vi "SendCom.vi"(8 "error in (no error)":errorcluster, 9 "data":variant, 10 "Command":T1="CONTROL:DAQmxConnect", 11 "Control in":refnum<class "Control-Server.lvclass">) -> (0 "error out":errorcluster, 3 "Control out":refnum<class "Control-Server.lvclass">)   [LabVIEW 2020, in "Control-Server.lvclass"]
uses:
  Control-Server.lvclass
  C:/dev/TRANCON/Classes/GeneralFunctionality/GeneralFunctionality.lvclass
  dependecies/ControlsVIs/Clusters-def/SERVER-Commands.ctl
  dependecies/ControlsVIs/Clusters-def/Message types.ctl
  Message/Message.lvclass
  GeneralFunctionality/GeneralFunctionality.lvclass
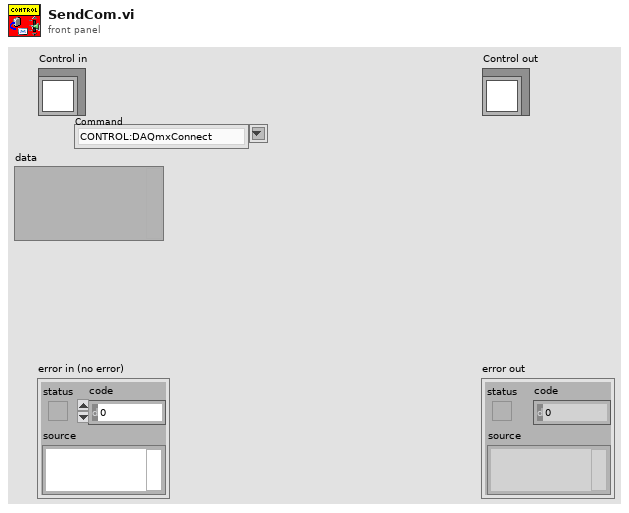
[diagram p1: front panel]
types:
  T1 = typedef "Control-Server.lvclass/SERVER-Commands.ctl" = string
  T2 = typedef "Message types.ctl" = string
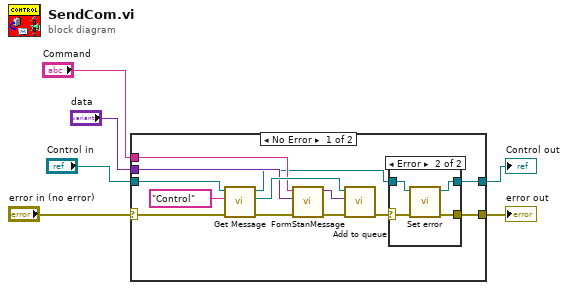
[diagram p0: block diagram]
diagram:
  n1 = case shown="No Error" "error in (no error)" {
    selector: "error in (no error)" -> [w19 w27]
    tunnel: [w16 w27] -> w5
    tunnel: [w8 w26] -> w3
    tunnel: "Control in" -> [w15 w26]
    tunnel: "Command" -> [w13 _]
    tunnel: "data" -> [w12 _]
    frame No Error {
      n2 = call "Get Message.vi"("error in (no error)"=w19, "Message type"=T2 "Control", "GeneralFunctionality en entrée"=w15) -> ("error out"=w11:errorcluster, "Message.lvclass"=w18:refnum<class "Message.lvclass">, "GeneralFunctionality en sortie"=w7:refnum<class "Control-Server.lvclass">)  [unwired: 6 in]
      n3 = call "FormStanMessage.vi"("error in"=w11, "data"=w12, "Command"=w13) -> ("error out"=w10:errorcluster, "message"=w14:variant)  [unwired: 7 in]
      n4 = call "Add to queue.vi"("error in (no error)"=w10, "Data"=w14, "Message in"=w18) -> ("error out"=w9:errorcluster)  [unwired: 7 in, 1 out]
      n5 = case shown="Error" w9 {
        selector: w9 -> [w20 w23]
        tunnel: [w20 w25] -> w16
        tunnel: w7 -> [w21 w24]
        tunnel: [w21 w22] -> w8
        frame No Error {
        }
        frame Error {
          n6 = call "Set error.vi"("error in (no error)"=w23, "Control-Server in"=w24) -> ("error out"=w25:errorcluster, "Control-Server out"=w22:refnum<class "Control-Server.lvclass">)  [unwired: 8 in]
        }
      }
    }
    frame Error {
    }
  }
  "error out" <- w5
  "Control out" <- w3
